vi "KVMap-From String.vi"(7 "delimiter (Tab)":string=":", 11 "value":string) -> (3 "Cluster":cluster{string[], string[]})   [LabVIEW 2012]
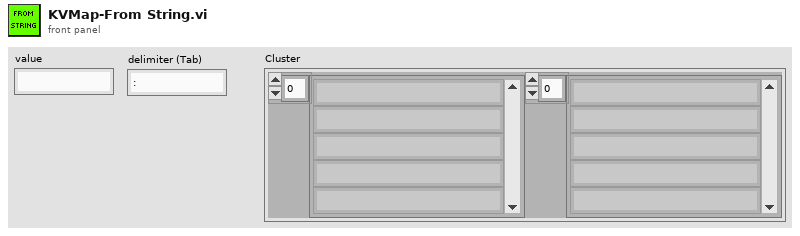
[diagram p1: front panel]
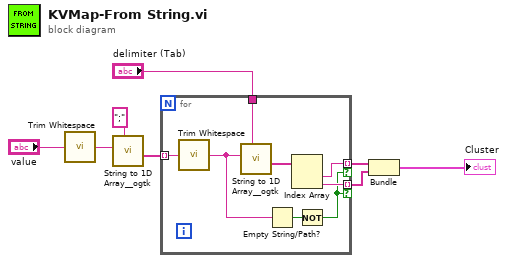
[diagram p0: block diagram]
diagram:
  n1 = call <vilib>:"Trim Whitespace.vi"("string"="value") -> ("trimmed string"=w5:string)  [unwired: 1 in]
  n2 = call <userlib>:"String to 1D Array__ogtk.vi"("delimiter (Tab)"=";", "string"=w5) -> ("Array of Strings"=w4:string[])  [unwired: 9 in]
  n3 = for {
    tunnel: w4 -> [w13] mode=indexing
    tunnel: [w15] -> w6 mode=indexing if=w10
    tunnel: [w14] -> w7 mode=indexing if=w10
    tunnel: "delimiter (Tab)" -> [w9]
    n4 = call <vilib>:"Trim Whitespace.vi"("string"=w13) -> ("trimmed string"=w12:string)  [unwired: 1 in]
    n5 = call <userlib>:"String to 1D Array__ogtk.vi"("delimiter (Tab)"=w9, "string"=w12) -> ("Array of Strings"=w16:string[])  [unwired: 9 in]
    n6 = Empty String/Path?(string/path=w12) -> (empty?=w11:bool)
    n7 = Index Array(array=w16) -> (element #1=w15:string, element #2=w14:string)  [unwired: 2 in]
    n8 = Not(x=w11) -> (.not. x?=w10:bool)
  }
  n9 = Bundle(w6, w7) -> (→"Cluster":cluster{string[], string[]})  [unwired: 1 in]
